vi "MeasureDetectorVoltage.vi"() -> (2 "Average Voltage":dbl)   [LabVIEW 2017]
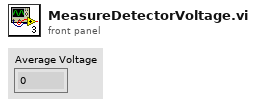
[diagram p1: front panel]
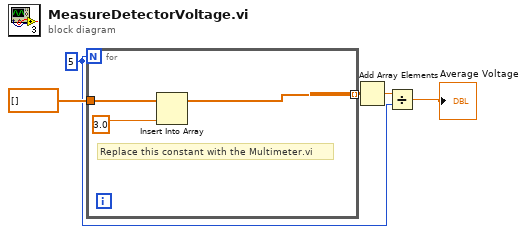
[diagram p0: block diagram]
diagram:
  w2 = 5
  n1 = for {
    N: w2 -> [_]
    tunnel: dbl[] [] ("array") -> [w8]
    tunnel: [w6] -> w4 mode=indexing
    # "Replace this constant with the Multimeter.vi"
    n2 = Insert Into Array(array=w8, new element=3.0) -> (w6:dbl[])  [unwired: 1 in]
  }
  n3 = Add Array Elements(numeric array=w4) -> (sum=w3:dbl)
  n4 = Divide(x=w3, y=w2) -> (x/y=→"Average Voltage":dbl)
